vi "Configure DC Input Resistance.vi"(8 "error in (no error)":errorcluster, 10 "Enable DC Input Resistance Mode (Enable)":bool=TRUE, 11 "VISA resource name":refnum<visa-resource-name>) -> (0 "error out":errorcluster, 3 "VISA resource name out":refnum<visa-resource-name>)   [LabVIEW 2013, in "Agilent 3458.lvlib"]
doc: "Configures the input resistance of the DMM to a constant 10 megaOhms. This applies to DC voltage measurements."
uses:
  Agilent 3458.lvlib
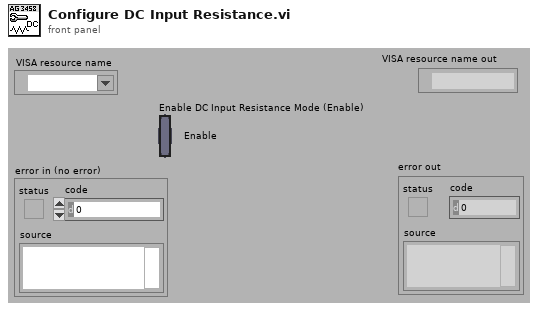
[diagram p1: front panel]
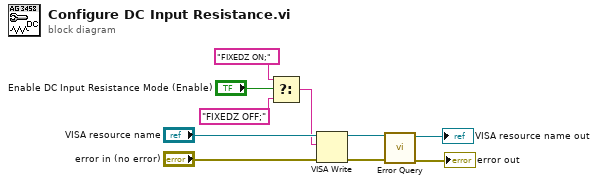
[diagram p0: block diagram]
diagram:
  n1 = Select(t="FIXEDZ ON;", s="Enable DC Input Resistance Mode (Enable)", f="FIXEDZ OFF;") -> (s? t:f=w2:string)
  n2 = VISA Write(VISA resource name="VISA resource name", write buffer=w2, error in (no error)="error in (no error)") -> (VISA resource name out=w9:refnum<visa-resource-name>, error out=w10:errorcluster)  [unwired: 1 out]
  n3 = call "Error Query.vi"("error in (no error)"=w10, "VISA resource name"=w9) -> ("error out"=→"error out":errorcluster, "VISA resource name out"=→"VISA resource name out":refnum<visa-resource-name>)  [unwired: 6 in, 2 out]
